vi "ChangeTimerPeroid.vi"(8 "error in (no error)":errorcluster, 9 "TimePeroid(ms)":i64, 10 "Name":string, 11 "TimerEngine in":refnum<class "TimerEngine.lvclass">) -> (0 "error out":errorcluster, 3 "TimerEngine out":refnum<class "TimerEngine.lvclass">)   [LabVIEW 2017, in "TimerEngine.lvlib" / "TimerEngine.lvclass"]
uses:
  TimerEngine.lvclass
  TimerEngine.lvclass/TimerEngine.ctl
  _TimerClass/Timer.lvclass/Timer.ctl
  _TimerClass/Timer.lvclass
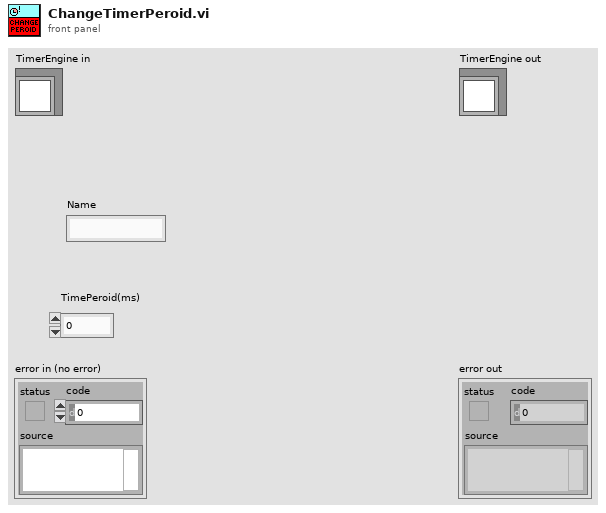
[diagram p1: front panel]
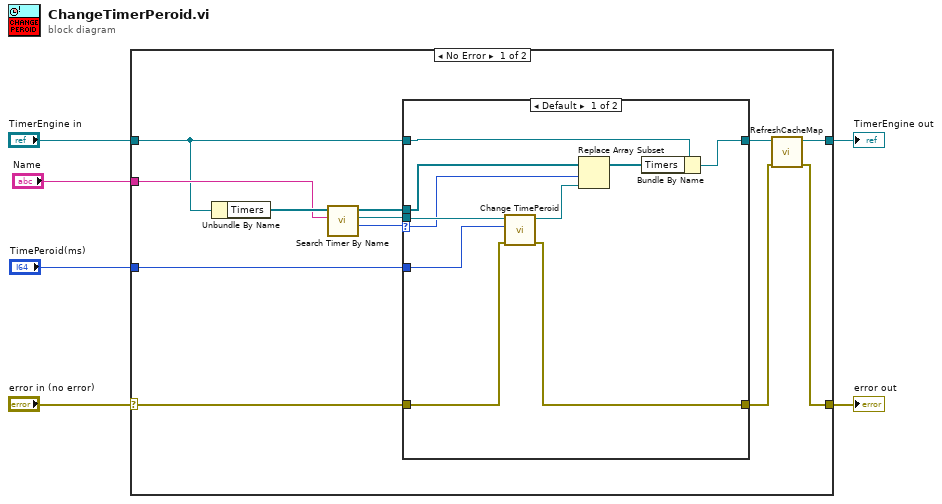
[diagram p0: block diagram]
diagram:
  n1 = case shown="No Error" "error in (no error)" {
    selector: "error in (no error)" -> [w13 w32]
    tunnel: [w7 w32] -> w5
    tunnel: [w9 w31] -> w3
    tunnel: "TimerEngine in" -> [w11 w31]
    tunnel: "Name" -> [w17 _]
    tunnel: "TimePeroid(ms)" -> [w15 _]
    frame No Error {
      n2 = Unbundle By Name(w11) -> ("Timers"=w18:refnum<class "Timer.lvclass">[])
      n3 = call "Search Timer By Name.vi"("Name"=w17, "Array"=w18) -> ("index of element"=w16:i32, "element"=w14:refnum<class "Timer.lvclass">, "Array 2"=w10:refnum<class "Timer.lvclass">[])  [unwired: 6 in, 1 out]
      n4 = case shown="Default" w16 {
        selector: w16 -> [w20 _]
        tunnel: w15 -> [w19 _]
        tunnel: w14 -> [w28 _]
        tunnel: w13 -> [w27 w30]
        tunnel: [w26 w30] -> w8
        tunnel: [w23 w29] -> w12
        tunnel: w11 -> [w25 w29]
        tunnel: w10 -> [w24 _]
        frame Default {
          n5 = call "Change TimePeroid.vi"("error in (no error)"=w27, "TimePeroid(ms)"=w19, "Timer in"=w28) -> ("error out"=w26:errorcluster, "Timer out"=w21:refnum<class "Timer.lvclass">)  [unwired: 7 in]
          n6 = Replace Array Subset(array=w24, new element=w21, index=w20) -> (w22:refnum<class "Timer.lvclass">[])
          n7 = Bundle By Name(cluster=w25, "Timers"=w22) -> (w23:refnum<class "TimerEngine.lvclass">)
        }
        frame -1 {
        }
      }
      n8 = call "RefreshCacheMap.vi"("error in (no error)"=w8, "UserEventTimer in"=w12) -> ("error out"=w7:errorcluster, "UserEventTimer out"=w9:refnum<class "TimerEngine.lvclass">)  [unwired: 8 in]
    }
    frame Error {
    }
  }
  "error out" <- w5
  "TimerEngine out" <- w3
